vi "Teardown.vi"(11 "Notifier Transport in":refnum<class "Notifier Transport.lvclass">) -> (2 "Unhandled Msgs":refnum<class "Msg.lvclass">[](array[class]))   [LabVIEW 2025, in "jettl.lvlib" / "Transport.lvlib" / "Notifier.lvlib" / "Notifier Transport.lvclass"]
uses:
  Notifier Transport.lvclass
  Notifier Transport.lvclass/Notifier Transport.ctl
  Msg/Msg.lvclass
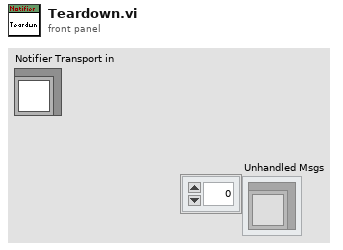
[diagram p1: front panel]
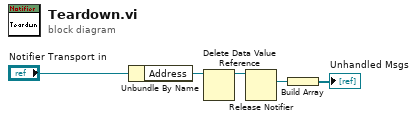
[diagram p0: block diagram]
diagram:
  n1 = Unbundle By Name("Notifier Transport in") -> ("Address"=w5:refnum<data-value>)
  n2 = Delete Data Value Reference(data value reference=w5) -> (data value=w3:refnum<notifier>)  [unwired: 1 in, 1 out]
  n3 = Release Notifier(notifier=w3) -> (last notification=w1:refnum<class "Msg.lvclass">)  [unwired: 2 in, 2 out]
  n4 = Build Array(w1) -> (→"Unhandled Msgs":refnum<class "Msg.lvclass">[])
